vi "Read Config File.vi"(8 "error in":errorcluster, 9 "keys":string[](array[string]), 10 "section":string, 11 "configuration file path":path) -> (0 "error out":errorcluster, 3 "Values":string[](array[string]))   [LabVIEW 2023]
uses:
  <vilib>/Utility/config.llb/Read Key (String).vi
  <vilib>/Utility/config.llb/NI_LVConfig.lvlib
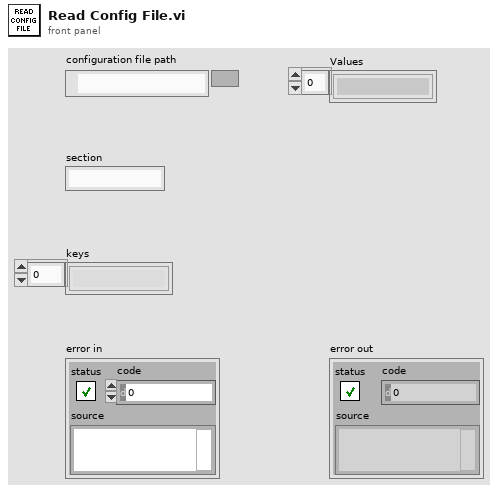
[diagram p1: front panel]
types:
  T1 = typedef "NI_LVConfig.lvlib/Config Data RefNum.ctl" = refnum<k1>
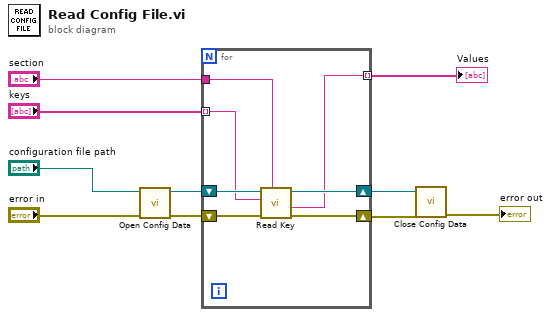
[diagram p0: block diagram]
diagram:
  n1 = call <vilib>:"Open Config Data.vi"("error in (no error)"="error in", "configuration file path"="configuration file path") -> ("error out"=w7:errorcluster, "refnum"=w8:T1)  [unwired: 7 in, 1 out]
  n2 = for {
    tunnel: "keys" -> [w15] mode=indexing
    tunnel: "section" -> [w14]
    shift-right: [w13] -> w4
    shift-left: w8 -> [w17]
    shift-right: [w12] -> w3
    shift-left: w7 -> [w16]
    tunnel: [w11] -> w1 mode=indexing
    n3 = call-poly <vilib>:"Read Key.vi"("section"=w14, "error in (no error)"=w16, "key"=w15, "refnum"=w17) -> ("error out"=w12:errorcluster, "value"=w11:string, "refnum out"=w13:T1)  [unwired: 4 in, 1 out]
  }
  "Values" <- w1
  n4 = call <vilib>:"Close Config Data.vi"("error in (no error)"=w3, "refnum"=w4) -> ("error out"=→"error out":errorcluster)  [unwired: 8 in, 1 out]
